vi "Logger_FGV.vi"(8 "error in (no error)":errorcluster caption="错误输入（无错误）", 11 "Logger 输入":refnum<class "Logger.lvclass">) -> (0 "error out":errorcluster caption="错误输出", 3 "Logger 输出":refnum<class "Logger.lvclass">)   [LabVIEW 2019, in "Logger.lvclass"]
uses:
  <userlib>/Logger/Logger.lvclass
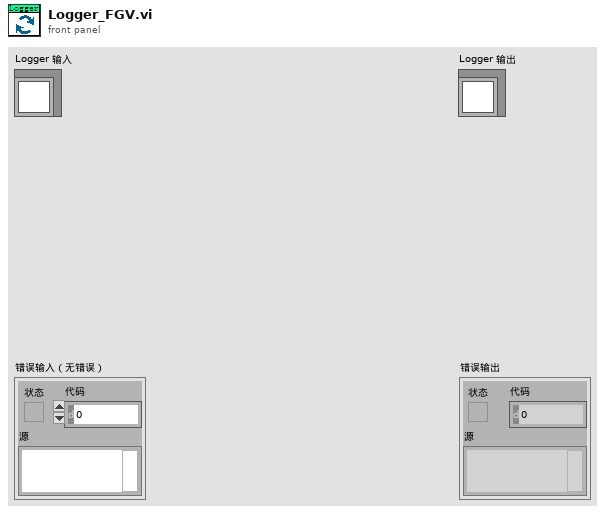
[diagram p1: front panel]
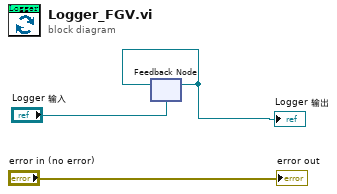
[diagram p0: block diagram]
diagram:
  n1 = feedback #1("Logger 输入") -> (w1:refnum<class "Logger.lvclass">)
  "Logger 输出" <- w1
  n2 = feedback-in #1(w1) -> ()
  "error out" <- "error in (no error)"
